vi "USRP_RXInit.vi"(0 "device names":refnum<k15>, 1 "USRP ControledParameters":T1={"active antenna"="TX1", "gain"=0.0, "carrier frequency"=100000.0, "IQ rate"=100000.0} {"IQ rate" format="%#_6p"; "carrier frequency" format="%#_6p"; "gain" format="%#_6f"}, 3 "error in (no error)":errorcluster) -> (7 "session handle out":refnum<k15>, 8 "USRP CoercedParamters":T2={"coerced IQ rate"=100000.0, "coerced carrier frequency"=100000.0, "coerced gain"=0.0} {"coerced gain" format="%#_6f"; "coerced carrier frequency" format="%#_6p"; "coerced IQ rate" format="%#_6p"}, 10 "error out":errorcluster)   [LabVIEW 2018]
panel:
  out "gain":dbl
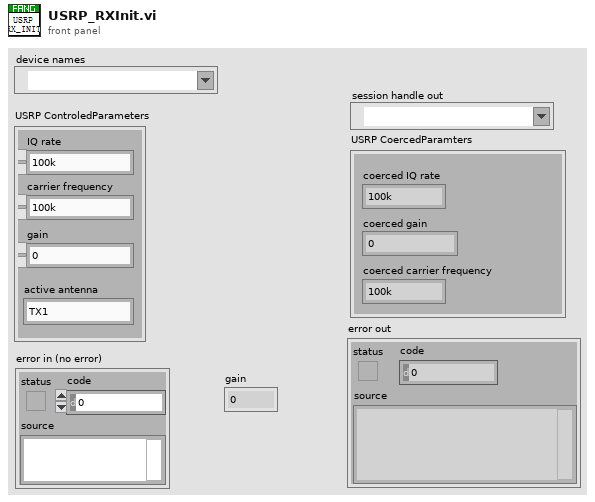
[diagram p1: front panel]
types:
  T1 = cluster{"active antenna":string, "gain":dbl, "carrier frequency":dbl, "IQ rate":dbl}
  T2 = cluster{"coerced IQ rate":dbl, "coerced carrier frequency":dbl, "coerced gain":dbl}
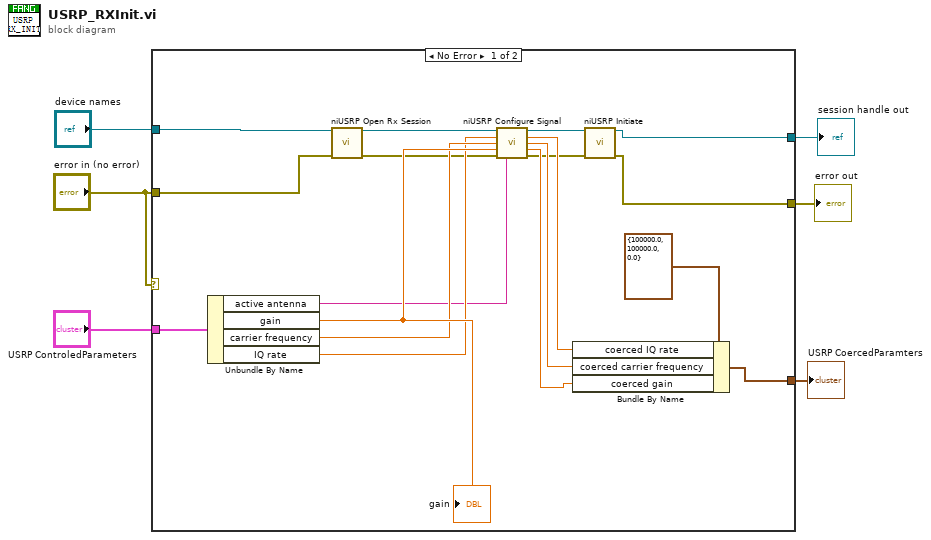
[diagram p0: block diagram]
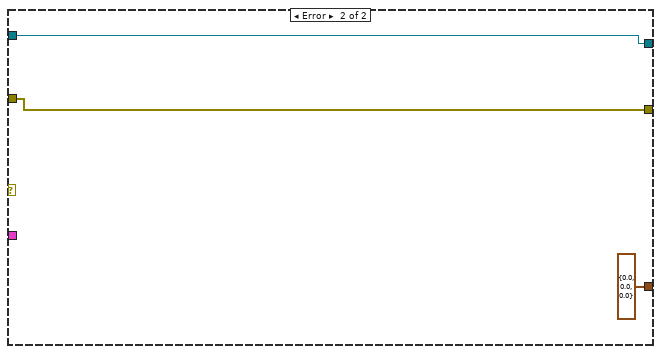
[diagram p2: hidden frame]
diagram:
  n1 = case shown="No Error" "error in (no error)" {
    tunnel: [w21 T2 {"coerced IQ rate"=0.0, "coerced carrier frequency"=0.0, "coerced gain"=0.0} ("USRP CoercedParamters")] -> w6
    tunnel: "USRP ControledParameters" -> [w16 _]
    tunnel: "device names" -> [w15 w26]
    tunnel: "error in (no error)" -> [w13 w27]
    tunnel: [w10 w27] -> w3
    tunnel: [w9 w26] -> w2
    frame No Error {
      n2 = Unbundle By Name(w16) -> ("active antenna"=w7:string, "gain"=w24:dbl, "carrier frequency"=w23:dbl, "IQ rate"=w22:dbl)
      "gain" <- w24
      n3 = call <instrlib>:"niUSRP Open Rx Session.vi"("device names"=w15, "error in (no error)"=w13) -> ("session handle out"=w14:refnum<k15>, "error out"=w12:errorcluster)  [unwired: 12 in]
      n4 = call <instrlib>:"niUSRP Configure Signal.vi"("session handle"=w14, "IQ rate"=w22, "carrier frequency"=w23, "gain"=w24, "error in (no error)"=w12, "active antenna"=w7) -> ("session handle out"=w8:refnum<k15>, "coerced IQ rate"=w20:dbl, "coerced carrier frequency"=w19:dbl, "coerced gain"=w18:dbl, "error out"=w11:errorcluster)  [unwired: 5 in]
      n5 = Bundle By Name(cluster=T2 {"coerced IQ rate"=100000.0, "coerced carrier frequency"=100000.0, "coerced gain"=0.0} ("USRP CoercedParamters"), "coerced IQ rate"=w20, "coerced carrier frequency"=w19, "coerced gain"=w18) -> (w21:T2)
      n6 = call <instrlib>:"niUSRP Initiate.vi"("session handle"=w8, "error in (no error)"=w11) -> ("session handle out"=w9:refnum<k15>, "error out"=w10:errorcluster)  [unwired: 12 in]
    }
    frame Error {
    }
  }
  "session handle out" <- w2
  "error out" <- w3
  "USRP CoercedParamters" <- w6
